vi "Remove Blanks.vi"(1 "INPUT STRING ARRAY":string[](array[string])) -> (0 "OUTPUT STRING ARRAY":string[](array[string]))   [LabVIEW 2015]
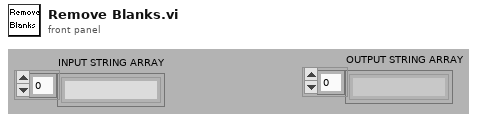
[diagram p1: front panel]
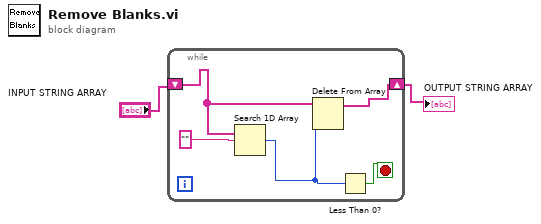
[diagram p0: block diagram]
diagram:
  n1 = while {
    shift-left: "INPUT STRING ARRAY" -> [w4]
    shift-right: [w3] -> w1
    stop <- w5 stop-if-true
    n2 = Search 1D Array(1D array=w4, element="") -> (index of element=w6:i32)  [unwired: 1 out]
    n3 = Delete From Array(array=w4, index=w6) -> (array with subset deleted=w3:string[])  [unwired: 1 in, 1 out]
    n4 = Less Than 0?(x=w6) -> (x < 0?=w5:bool)
  }
  "OUTPUT STRING ARRAY" <- w1
